vi "MySQL_Close_DB.vi"(8 "Status/Errors in":refnum<vi>, 11 "Write Data Parameters in":T1 {"Data storage"."Detector number" format="%#.0f"}) -> (0 "Status/Errors out":refnum<vi>, 3 "Write Data Parameters out":T1 {"Data storage"."Detector number" format="%#.0f"})   [LabVIEW 2010]
doc: "Closes the connection with the database (if there ever was a connection)."
uses:
  Controls/Write_Data_Parameters.ctl
  Controls/Stop_Loop.ctl
  Controls/Data_Storage.ctl
  Controls/DB_Connection.ctl
  database/Connection.llb/Conn ObjectReference.ctl
  Controls/Data_Storage_Condition.ctl
  Controls/GPS_Timestamp.ctl
  Controls/Get_Set_Statistics_Options2.ctl
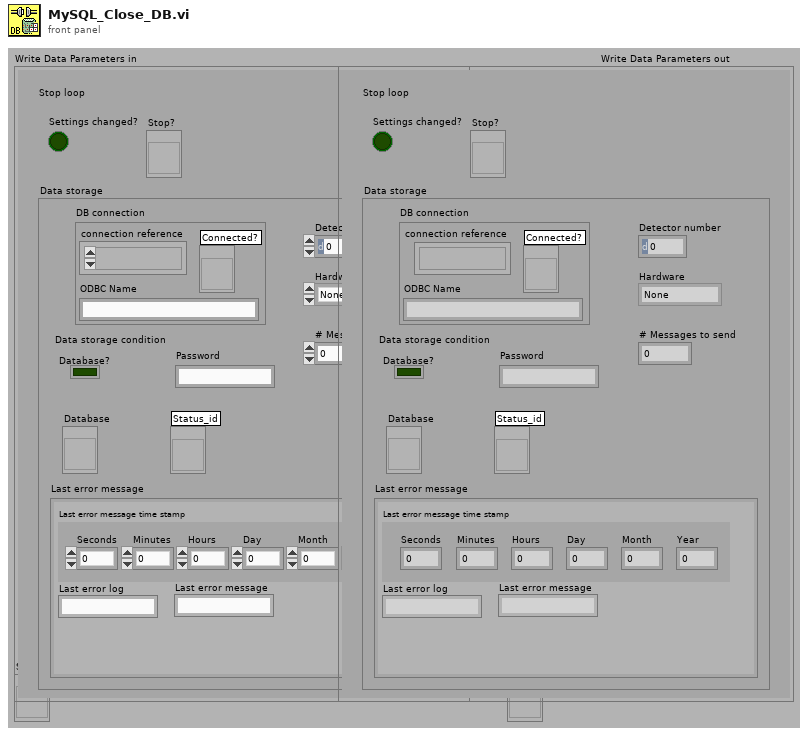
[diagram p1: front panel]
types:
  T1 = typedef "Write_Data_Parameters.ctl" = cluster{"Stop loop":T2, "Data storage":T3}
  T2 = typedef "Stop_Loop.ctl" = cluster{"Settings changed?":bool, "Stop?":refnum<vi>}
  T3 = typedef "Data_Storage.ctl" = cluster{"DB connection":T4, "Data storage condition":T6, "Detector number":u16, "# Messages to send":i32, "Database":refnum<vi>, "Password":string, "Last error message":cluster{"Last error message time stamp":T7, "Last error log":string, "Last error message":string}, "Status_id":refnum<vi>, "Hardware":enum8{"None", "HiSPARC I", "HiSPARC II", "HiSPARC III", "Unknown"}}
  T4 = typedef "DB_Connection.ctl" = cluster{"connection reference":T5, "Connected?":refnum<vi>, "ODBC Name":string}
  T5 = typedef "Conn ObjectReference.ctl" = refnum<k1>
  T6 = typedef "Data_Storage_Condition.ctl" = cluster{"Database?":bool}
  T7 = typedef "GPS_Timestamp.ctl" = cluster{"Seconds":u8, "Minutes":u8, "Hours":u8, "Day":u8, "Month":u8, "Year":u16}
  T8 = typedef "Get_Set_Statistics_Options2.ctl" = enum16{"Get", "Set"}
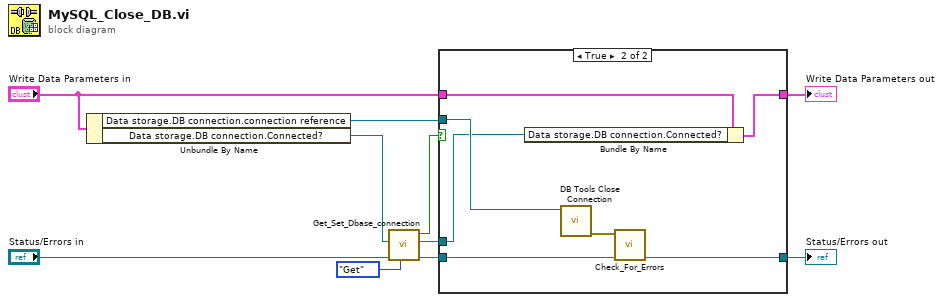
[diagram p0: block diagram]
diagram:
  n1 = Unbundle By Name("Write Data Parameters in") -> ("Data storage.DB connection.connection reference"=w10:T5, "Data storage.DB connection.Connected?"=w5:refnum<vi>)
  n2 = call "Get_Set_Dbase_connection.vi"("Get/Set"=Get_Set_Statistics_Options2."Get", "Status/Errors in"="Status/Errors in", "Connected? in"=w5) -> ("Status/Errors out"=w2:refnum<vi>, "Connected? out"=w1:refnum<vi>, "Value out"=w6:bool)  [unwired: 1 in, 5 out]
  n3 = case shown="True" w6 {
    tunnel: w10 -> [_ w18]
    tunnel: "Write Data Parameters in" -> [w11 w19]
    tunnel: w2 -> [w12 w17]
    tunnel: [w12 w16] -> w9
    tunnel: [w11 w14] -> w7
    tunnel: w1 -> [_ w13]
    frame False {
    }
    frame True {
      n4 = Bundle By Name(cluster=w19, "Data storage.DB connection.Connected?"=w13) -> (w14:T1)
      n5 = call "DB Tools Close Connection.vi"("connection reference"=w18) -> ("error out"=w15:errorcluster)  [unwired: 1 in, 5 out]
      n6 = call "Check_For_Errors.vi"("Status/Errors in"=w17, "error in"=w15) -> ("Status/Errors out"=w16:refnum<vi>)  [unwired: 9 out]
    }
  }
  "Status/Errors out" <- w9
  "Write Data Parameters out" <- w7
